vi "sub FM0decode.vi"(10 "threshold":i32=3, 11 "Bit Sequence":i16[](array[numeric])) -> (3 "RN16 array":i32[](array[numeric]))   [LabVIEW 2015]
doc: "This example shows how the Write to Text File and Read from Text File functions operate using different options."
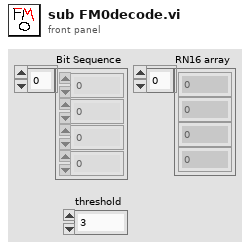
[diagram p1: front panel]
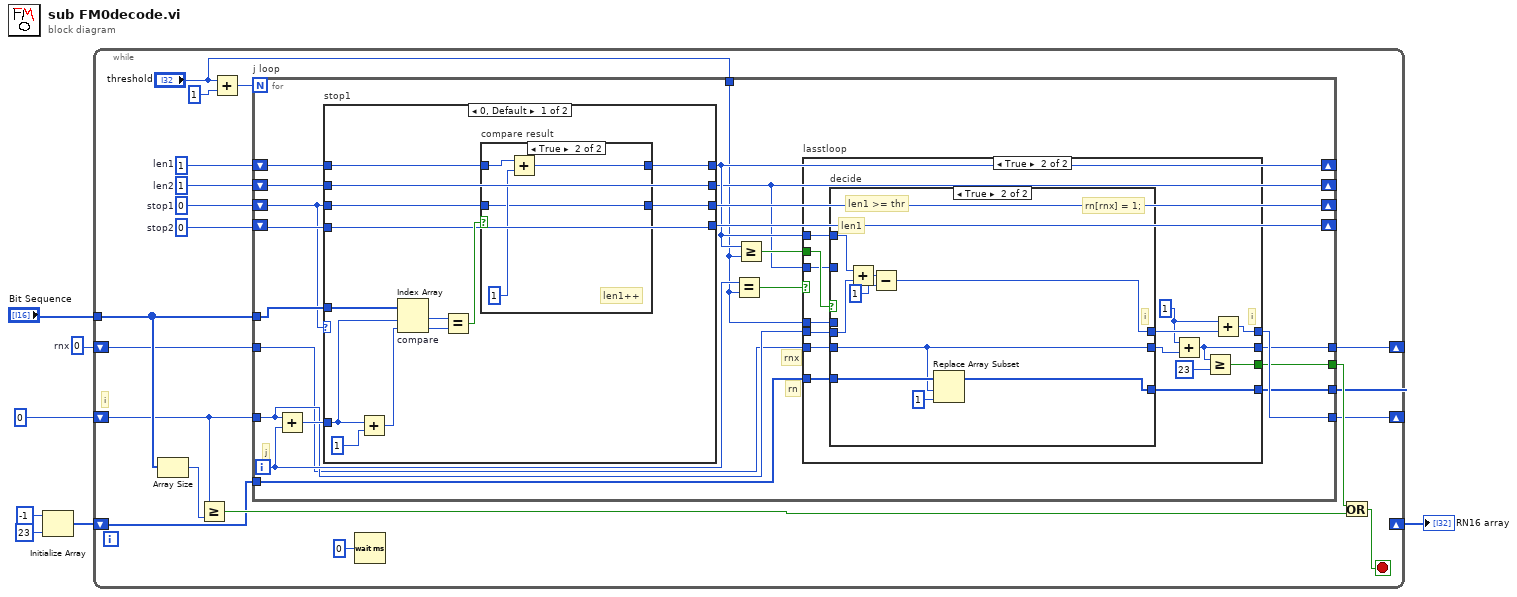
[diagram p0: block diagram]
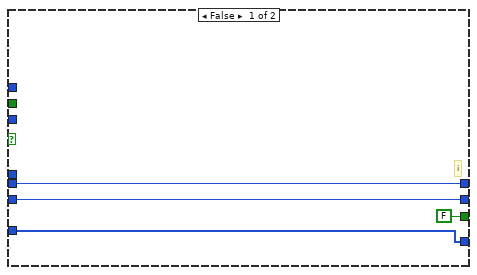
[diagram p2: hidden frame]
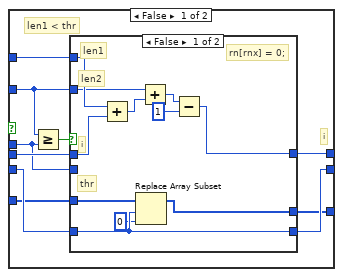
[diagram p3: hidden frame]
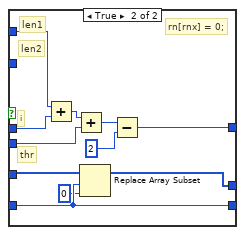
[diagram p4: hidden frame]
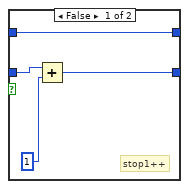
[diagram p5: hidden frame]
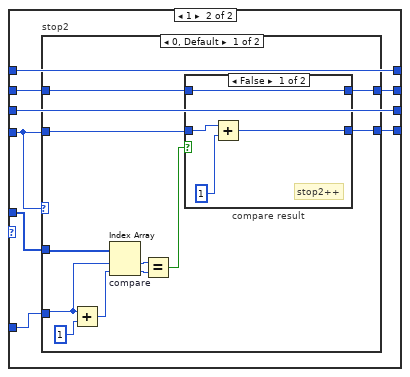
[diagram p6: hidden frame]
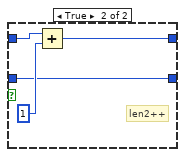
[diagram p7: hidden frame]
diagram:
  w7 = 0  # rnx
  n1 = Initialize Array(-1 ("element"), 23 ("dimension size")) -> (w5:i32[])
  n2 = while {
    tunnel: "Bit Sequence" -> [w22]
    shift-right: [w10] -> _
    shift-left: 0 -> [w11]
    shift-right: [w13] -> _
    shift-left: w7 -> [w12]
    shift-right: [w8] -> w2
    shift-left: w5 -> [w9]
    stop <- w19 stop-if-true
    w26 = 0  # stop2
    w25 = 0  # stop1
    w24 = 1  # len2
    w23 = 1  # len1
    # "i"
    n3 = Array Size(array=w22) -> (size(s)=w21:i32)
    n4 = Greater Or Equal?(x=w11, y=w21) -> (x >= y?=w18:bool)
    n5 = Add(x="threshold", y=1) -> (x+y=w15:i32)
    n6 = for "j loop" {
      N: w15 -> [_]
      tunnel: w22 -> [w43]
      shift-right: [w35] -> _
      shift-left: w23 -> [w47]
      shift-right: [w41] -> _
      shift-left: w25 -> [w42]
      shift-right: [w40] -> _
      shift-left: w26 -> [w45]
      shift-right: [w31] -> _
      shift-left: w24 -> [w46]
      tunnel: "threshold" -> [w29]
      tunnel: [w30] -> w20
      tunnel: w11 -> [w36]
      tunnel: [w34] -> w10
      tunnel: w12 -> [w33]
      tunnel: [w32] -> w13
      tunnel: w9 -> [w28]
      tunnel: [w27] -> w8
      i -> [w39]
      # "rn"
      # "rnx"
      # "j"
      n7 = Add(x=w36, y=w39) -> (x+y=w44:i32)
      n8 = case "stop1" shown="0, Default" w42 {
        tunnel: w47 -> [w113 w136]
        tunnel: w46 -> [w109 w131]
        tunnel: w45 -> [w108 w133]
        tunnel: w44 -> [w119 w129]
        tunnel: w43 -> [w117 w134]
        tunnel: [w112 w136] -> w35
        tunnel: w42 -> [w111 w135]
        tunnel: [w110 w135] -> w41
        tunnel: [w108 w132] -> w40
        tunnel: [w109 w130] -> w31
        frame 0, Default {
          n9 = Add(x=w119, y=1) -> (x+y=w120:i32)
          n10 = Index Array "compare"(array=w117, index #1=w119, index #2=w120) -> (element #1=w115:i16, element #2=w116:i16)
          n11 = Equal?(x=w115, y=w116) -> (x = y?=w114:bool)
          n12 = case "compare result" shown="True" w114 {
            tunnel: w113 -> [w124 w128]
            tunnel: [w124 w127] -> w112
            tunnel: w111 -> [w122 w125]
            tunnel: [w123 w125] -> w110
            frame False {
              # "stop1++"
              n13 = Add(x=w122, y=1) -> (x+y=w123:i32)
            }
            frame True {
              # "len1++"
              n14 = Add(x=w128, y=1) -> (x+y=w127:i32)
            }
          }
        }
        frame 1 {
          n15 = case "stop2" shown="0, Default" w133 {
            tunnel: w134 -> [w144 _]
            tunnel: w133 -> [w143 w156]
            tunnel: [w142 w156] -> w132
            tunnel: w131 -> [w141 w157]
            tunnel: [w140 w157] -> w130
            tunnel: w129 -> [w137 _]
            frame 0, Default {
              n16 = Add(x=w137, y=1) -> (x+y=w145:i32)
              n17 = Index Array "compare"(array=w144, index #1=w137, index #2=w145) -> (element #1=w147:i16, element #2=w146:i16)
              n18 = Equal?(x=w147, y=w146) -> (x = y?=w138:bool)
              n19 = case "compare result" shown="False" w138 {
                tunnel: w141 -> [w151 w155]
                tunnel: [w151 w154] -> w140
                tunnel: w143 -> [w149 w152]
                tunnel: [w150 w152] -> w142
                frame False {
                  # "stop2++"
                  n20 = Add(x=w149, y=1) -> (x+y=w150:i32)
                }
                frame True {
                  # "len2++"
                  n21 = Add(x=w155, y=1) -> (x+y=w154:i32)
                }
              }
            }
            frame 1 {
            }
          }
        }
      }
      n22 = Equal?(x=w39, y=w29) -> (x = y?=w38:bool)
      n23 = Greater Or Equal?(x=w35, y=w29) -> (x >= y?=w37:bool)
      n24 = case "lasstloop" shown="True" w38 {
        tunnel: w37 -> [_ w64]
        tunnel: w36 -> [w51 w66]
        tunnel: w35 -> [_ w65]
        tunnel: [w51 w57] -> w34
        tunnel: w33 -> [w50 w55]
        tunnel: [w50 w62] -> w32
        tunnel: w31 -> [_ w63]
        tunnel: [FALSE w60] -> w30
        tunnel: w29 -> [_ w59]
        tunnel: w28 -> [w48 w53]
        tunnel: [w48 w52] -> w27
        frame False {
          # "i"
        }
        frame True {
          w56 = 1 ("y")
          # "i"
          n25 = case "decide" shown="True" w64 {
            tunnel: w66 -> [w76 w106]
            tunnel: w65 -> [w72 w107]
            tunnel: [w71 w104] -> w58
            tunnel: w63 -> [w74 _]
            tunnel: w59 -> [w73 _]
            tunnel: [w69 w100] -> w54
            tunnel: w55 -> [w70 w100]
            tunnel: w53 -> [w68 w102]
            tunnel: [w67 w101] -> w52
            frame False {
              # "i"
              # "len1 < thr"
              n26 = Greater Or Equal?(x=w74, y=w73) -> (x >= y?=w75:bool)
              n27 = case shown="False" w75 {
                tunnel: w74 -> [w84 _]
                tunnel: w76 -> [w86 w97]
                tunnel: w73 -> [_ w95]
                tunnel: w72 -> [w87 w98]
                tunnel: [w81 w92] -> w71
                tunnel: [w79 w89] -> w69
                tunnel: w70 -> [w79 w89]
                tunnel: w68 -> [w80 w91]
                tunnel: [w77 w90] -> w67
                frame False {
                  # "rn[rnx] = 0;"
                  # "thr"
                  # "len2"
                  # "i"
                  # "len1"
                  n28 = Add(x=w87, y=w86) -> (x+y=w85:i32)
                  n29 = Replace Array Subset(array=w80, new element=0 ("new element/subarray"), index=w79) -> (w77:i32[])
                  n30 = Add(x=w84, y=w85) -> (x+y=w83:i32)
                  n31 = Subtract(x=w83, y=1) -> (x-y=w81:i32)
                }
                frame True {
                  # "rn[rnx] = 0;"
                  # "len2"
                  # "thr"
                  # "i"
                  # "len1"
                  n32 = Add(x=w98, y=w97) -> (x+y=w96:i32)
                  n33 = Add(x=w96, y=w95) -> (x+y=w94:i32)
                  n34 = Replace Array Subset(array=w91, new element=0 ("new element/subarray"), index=w89) -> (w90:i32[])
                  n35 = Subtract(x=w94, y=2) -> (x-y=w92:i32)
                }
              }
            }
            frame True {
              # "rn[rnx] = 1;"
              # "len1"
              # "i"
              # "len1 >= thr"
              n36 = Add(x=w107, y=w106) -> (x+y=w105:i32)
              n37 = Subtract(x=w105, y=1) -> (x-y=w104:i32)
              n38 = Replace Array Subset(array=w102, new element=1 ("new element/subarray"), index=w100) -> (w101:i32[])
            }
          }
          n39 = Add(x=w56, y=w54) -> (x+y=w62:i32)
          n40 = Greater Or Equal?(x=w62, y=23) -> (x >= y?=w60:bool)
          n41 = Add(x=w56, y=w58) -> (x+y=w57:i32)
        }
      }
    }
    n42 = Wait (ms)(milliseconds to wait=u32 0) -> ()  [unwired: 1 out]
    n43 = Or(x=w20, y=w18) -> (x .or. y?=w19:bool)
  }
  "RN16 array" <- w2
